vi "SetHandlerLevel.vi"(8 "error in (no error)":errorcluster, 9 "Level":T1=enum."WARNING", 10 "Handler in":refnum<class "Handler.lvclass">, 11 "Logger in":refnum<class "Logger.lvclass">) -> (0 "error out":errorcluster, 2 "Handler out":refnum<class "Handler.lvclass">, 3 "Logger out":refnum<class "Logger.lvclass">)   [LabVIEW 2022 SP3, in "Logger.lvlib" / "Logger.lvclass"]
uses:
  Logger.lvclass
  C:/Users/jakub/repos/gh/PythonWrapper/Source/PythonWrapper/PythonWrapper.lvclass
  _Level.ctl
  PythonWrapper/Source/PythonWrapper/PythonWrapper.lvclass/PythonWrapper.ctl
  Logger.lvclass/Logger.ctl
  PythonWrapper/Source/PythonWrapper/Read PythonSession.vi
  PythonWrapper/Source/PythonWrapper/Read ModulePath.vi
  Handler/Handler.lvclass
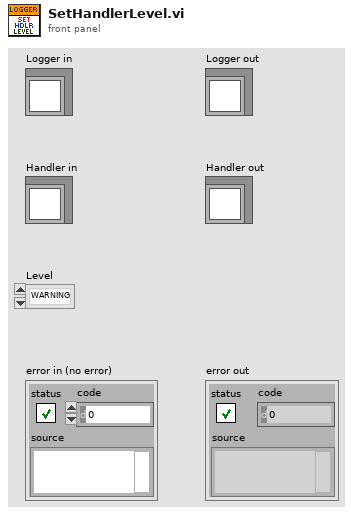
[diagram p1: front panel]
types:
  T1 = typedef "Logger.lvlib/Logger.lvclass/_Level.ctl" = enum16{"NOTSET", "DEBUG", "INFO", "WARNING", "ERROR", "CRITICAL"}
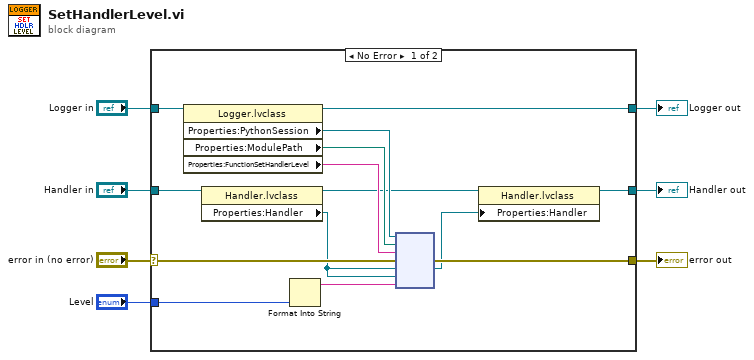
[diagram p0: block diagram]
diagram:
  n1 = case shown="No Error" "error in (no error)" {
    selector: "error in (no error)" -> [w19 w23]
    tunnel: [w18 w23] -> w4
    tunnel: [w20 w22] -> w5
    tunnel: "Logger in" -> [w21 w22]
    tunnel: "Level" -> [w14 _]
    tunnel: "Handler in" -> [w12 _]
    tunnel: [w8 _] -> w1
    frame No Error {
      n2 = property class="Logger.lvclass"(reference=w21) -> (reference out=w20:refnum<class "Logger.lvclass">, "Properties:PythonSession"=w17:refnum<k35>, "Properties:ModulePath"=w15:path, "Properties:FunctionSetHandlerLevel"=w16:string)  [unwired: 1 in, 1 out]
      n3 = property class="Handler.lvclass"(reference=w12) -> (reference out=w10:refnum<class "Handler.lvclass">, "Properties:Handler"=w11:refnum<k38>)  [unwired: 1 in, 1 out]
      n4 = Format Into String(w14) -> (resulting string=w13:string)  [unwired: 3 in, 1 out]
      n5 = node(w17, w15, w16, w19, w11, w11, w13) -> (w18:errorcluster, w9:refnum<k38>)  [unwired: 2 in, 3 out]
      n6 = property class="Handler.lvclass"(reference=w10, "Properties:Handler"=w9) -> (reference out=w8:refnum<class "Handler.lvclass">)  [unwired: 1 in, 1 out]
    }
    frame Error {
    }
  }
  "error out" <- w4
  "Logger out" <- w5
  "Handler out" <- w1
